vi "Test Base64URL Encoder and Decoder.vi"() -> ()   [LabVIEW 2013]
uses:
  <vilib>/LabVIEW Open Source Project/OpenSerializer/Serializer/Serializer.lvclass
  source-base64/Serializer.Base64.lvclass
panel:
  out "Decoded String 2":string
  out "Encoded String 2":string
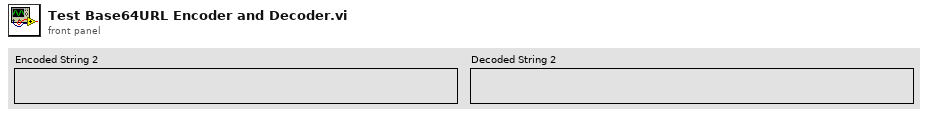
[diagram p1: front panel]
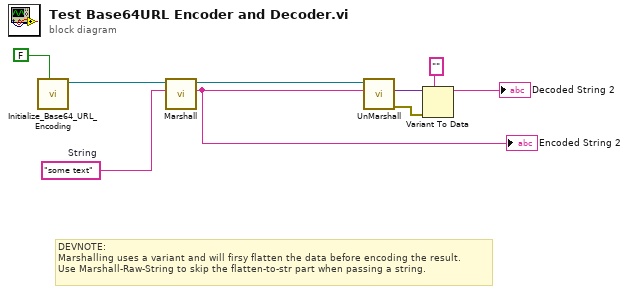
[diagram p0: block diagram]
diagram:
  w6 = "some text"  # String
  # "DEVNOTE: \nMarshalling uses a variant and will firsy flatten the data before encoding the result.\nUse Marshall-Raw-String to skip the flatten-to-str part when passing a string."
  n1 = call "Initialize_Base64_URL_Encoding.vi"("marshal-raw-string"=FALSE ("marshall-raw-string")) -> ("Base64 URL Encoding"=w8:refnum<class "Serializer.Base64.lvclass">)  [unwired: 10 in]
  n2 = call <vilib>:"Marshall.vi"("Variant"=w6, "Serializer in"=w8) -> ("String"=w7:string, "Serializer out"=w5:refnum<class "Serializer.Base64.lvclass">)  [unwired: 7 in, 1 out]
  "Encoded String 2" <- w7
  n3 = call <vilib>:"UnMarshall.vi"("String"=w7, "Serializer in"=w5) -> ("error out"=w1:errorcluster, "Variant"=w3:variant)  [unwired: 7 in, 1 out]
  n4 = Variant To Data(error in=w1, type="", Variant=w3) -> (data=→"Decoded String 2":string)  [unwired: 1 out]
